vi "Write Tttl.vi"(8 "error in (no error)":errorcluster, 10 "Tttl":string, 11 "Termination in":refnum<class "Termination.lvclass">) -> (0 "error out":errorcluster, 3 "Termination out":refnum<class "Termination.lvclass">)   [LabVIEW 2020, in "Termination.lvclass"]
uses:
  Termination.lvclass
  Termination.lvclass/Termination.ctl
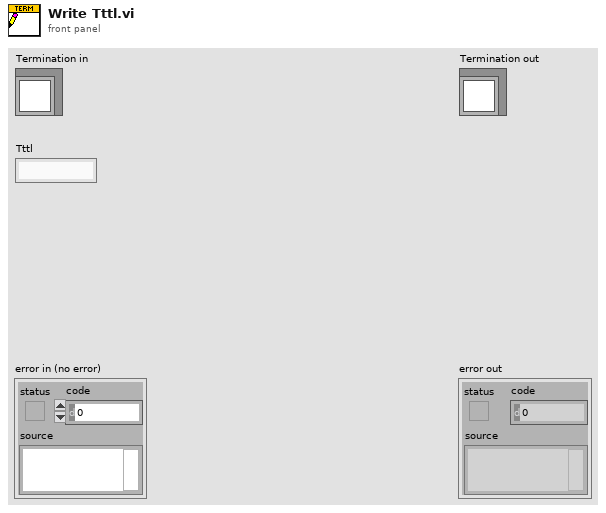
[diagram p1: front panel]
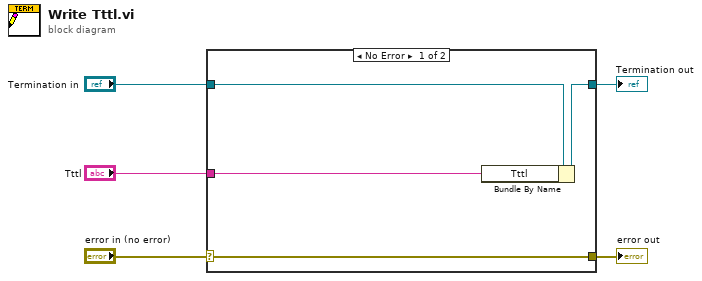
[diagram p0: block diagram]
diagram:
  n1 = case shown="No Error" "error in (no error)" {
    selector: "error in (no error)" -> [w9 w10]
    tunnel: [w9 w10] -> w4
    tunnel: [w7 w11] -> w2
    tunnel: "Termination in" -> [w8 w11]
    tunnel: "Tttl" -> [w6 _]
    frame No Error {
      n2 = Bundle By Name(cluster=w8, "Tttl"=w6) -> (w7:refnum<class "Termination.lvclass">)
    }
    frame Error {
    }
  }
  "error out" <- w4
  "Termination out" <- w2
